vi "CAN通信实验.vi"() -> ()   [LabVIEW 2011]
uses:
  <vilib>/STM32_DriverVI_Interface_F4/CAN/Frame Stand_Extend_F4.ctl
  <vilib>/STM32_DriverVI_Interface_F4/CAN/Frame Data_Remote_F4.ctl
  <vilib>/STM32_DriverVI_Interface_F4/CAN/CAN Mode Set_F4.ctl
  <vilib>/STM32_DriverVI_Interface_F4/CAN/CAN Baud Rate_F4.ctl
  <vilib>/STM32_DriverVI_Interface_F4/CAN/CAN1_TX Pin Map_F4.ctl
  <vilib>/STM32_DriverVI_Interface_F4/CAN/CAN1_RX Pin Map_F4.ctl
  <vilib>/STM32_DriverVI_Interface_F4/CAN/CAN Filter_X Set_F4.ctl
  <vilib>/STM32_DriverVI_Interface_F4/CAN/Filter Enable_F4.ctl
  <vilib>/STM32_DriverVI_Interface_F4/CAN/CAN1 Init_F4.vi
  <vilib>/STM32_DriverVI_Interface_F4/CAN/CAN1 Filter Set_F4.vi
  <vilib>/STM32_DriverVI_Interface_F4/CAN/CAN1 Send Frame_F4.vi
  <vilib>/STM32_DriverVI_Interface_F4/CAN/CAN1 Frame Count_F4.vi
  <vilib>/STM32_DriverVI_Interface_F4/CAN/CAN1 Read Frame_F4.vi
panel:
  out "Send Success？":u16
  out "Init Success？":bool
  out "Frame Counts":u16
  out "Frame_Data":u8[][](array[numeric])
  in  "是否读取":bool
  in  "Frame Data or Remote":T1
  in  "Frame Stand or Extend":T2
  in  "Frame_ID":u32
  in  "数组长度":i32
  in  "点击发送":bool
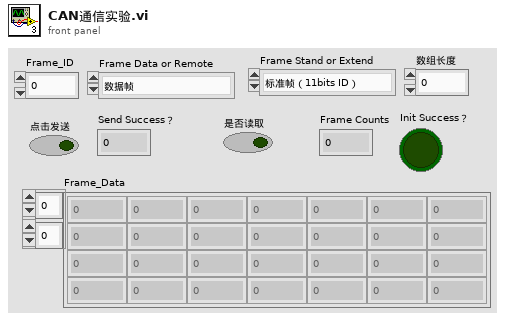
[diagram p1: front panel]
types:
  T1 = typedef "Frame Data_Remote_F4.ctl" = enum8{"数据帧", "远程帧"}
  T2 = typedef "Frame Stand_Extend_F4.ctl" = enum8{"标准帧（11bits ID）", "扩展帧（29bits ID）"}
  T3 = typedef "CAN Filter_X Set_F4.ctl" = enum8{"Filter_0", "Filter_1", "Filter_2", "Filter_3", "Filter_4", "Filter_5", "Filter_6", "Filter_7", "Filter_8", "Filter_9", "Filter_10", "Filter_11", "Filter_12", "Filter_13", "Filter_14", "Filter_15", "Filter_16", "Filter_17", "Filter_18", "Filter_19", "Filter_20", "Filter_21", "Filter_22", "Filter_23", "Filter_24", "Filter_25", "Filter_26", "Filter_27"}
  T4 = typedef "Filter Enable_F4.ctl" = enum8{"Disable", "Enable"}
  T5 = typedef "CAN1_RX Pin Map_F4.ctl" = u8
  T6 = typedef "CAN1_TX Pin Map_F4.ctl" = u8
  T7 = typedef "CAN Baud Rate_F4.ctl" = u16
  T8 = typedef "CAN Mode Set_F4.ctl" = enum8{"正常发送", "环回模式"}
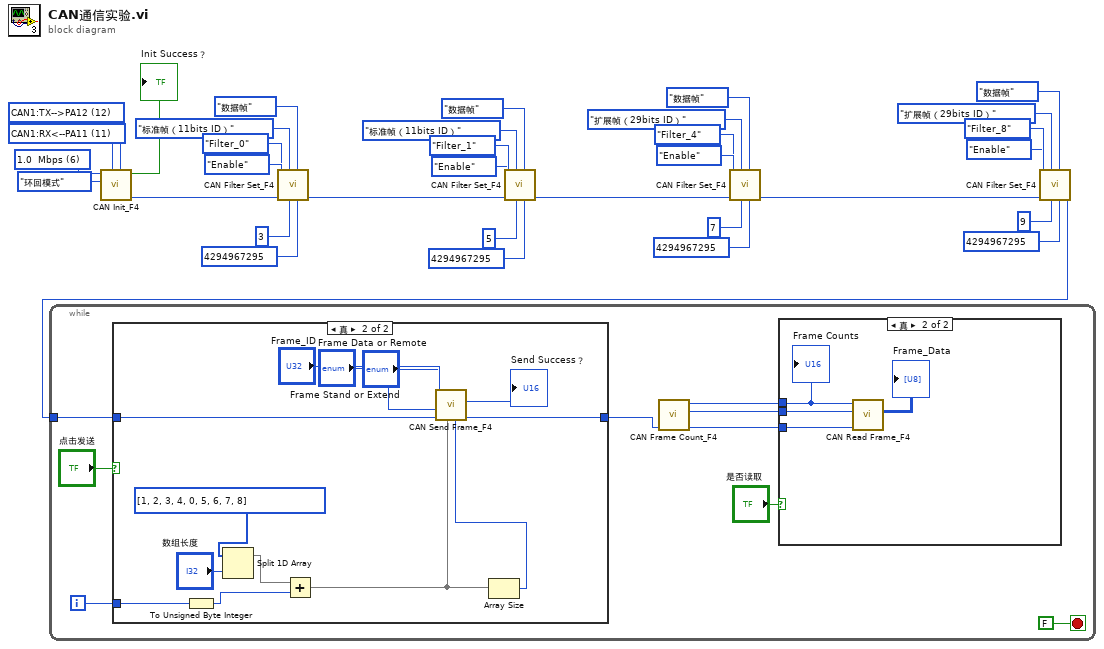
[diagram p0: block diagram]
diagram:
  w31 = T5 11 items=["CAN1:RX<--PA11"=11, "CAN1:RX<--PB8"=24, "CAN1:RX<--PD0"=48, "CAN1:RX<--PI9"=137] ("CAN1_RX Pin Map")
  w32 = T6 12 items=["CAN1:TX-->PA12"=12, "CAN1:TX-->PB9"=25, "CAN1:TX-->PD1"=49, "CAN1:TX-->PH13"=125] ("CAN1_TX Pin Map")
  w33 = T7 6 items=["1.0  Mbps"=6, "750 Kbps"=8, "600  Kbps"=10, "500  Kbps"=12, "400  Kbps"=15, "375  Kbps"=16, "300  Kbps"=20, "250  Kbps"=24, "200  Kbps"=30, "187.5Kbps"=32, "150   Kbps"=40, "125   Kbps"=48, "120   Kbps"=50, "100   Kbps"=60, "75     Kbps"=80, "60    Kbps"=100, "50    Kbps"=120, "40    Kbps"=150, "37.5  Kbps"=160, "30    Kbps"=200, "25    Kbps"=240, "20    Kbps"=300, "10    Kbps"=600, "5      Kbps"=1200] ("CAN Baud Rate")
  n1 = call-poly <vilib>:"CAN Init_F4.vi"("CAN1_RX Pin Map"=w31, "CAN1_TX Pin Map"=w32, "CAN Mode Setting"=CAN_Mode_Set_F4."环回模式", "CAN Baud Rate"=w33) -> ("err_out"=w30:u8, "Init Success？"=→"Init Success？":bool)  [unwired: 6 in]
  n2 = call-poly <vilib>:"CAN Filter Set_F4.vi"("ID_Mask"=u32 4294967295, "Frame Data or Remote"=Frame_Data_Remote_F4."数据帧", "Filter_ID"=u32 3, "Frame Stand or Extend"=Frame_Stand_Extend_F4."标准帧（11bits ID）", "err_in"=w30, "Filter Enable/Disable"=Filter_Enable_F4."Enable", "CAN Filter_X Setting"=CAN_Filter_X_Set_F4."Filter_0") -> ("err_out"=w5:u8)  [unwired: 4 in]
  n3 = call-poly <vilib>:"CAN Filter Set_F4.vi"("ID_Mask"=u32 4294967295, "Frame Data or Remote"=Frame_Data_Remote_F4."数据帧", "Filter_ID"=u32 5, "Frame Stand or Extend"=Frame_Stand_Extend_F4."标准帧（11bits ID）", "err_in"=w5, "Filter Enable/Disable"=Filter_Enable_F4."Enable", "CAN Filter_X Setting"=CAN_Filter_X_Set_F4."Filter_1") -> ("err_out"=w4:u8)  [unwired: 4 in]
  n4 = call-poly <vilib>:"CAN Filter Set_F4.vi"("ID_Mask"=u32 4294967295, "Frame Data or Remote"=Frame_Data_Remote_F4."数据帧", "Filter_ID"=u32 7, "Frame Stand or Extend"=Frame_Stand_Extend_F4."扩展帧（29bits ID）", "err_in"=w4, "Filter Enable/Disable"=Filter_Enable_F4."Enable", "CAN Filter_X Setting"=CAN_Filter_X_Set_F4."Filter_4") -> ("err_out"=w3:u8)  [unwired: 4 in]
  n5 = call-poly <vilib>:"CAN Filter Set_F4.vi"("ID_Mask"=u32 4294967295, "Frame Data or Remote"=Frame_Data_Remote_F4."数据帧", "Filter_ID"=u32 9, "Frame Stand or Extend"=Frame_Stand_Extend_F4."扩展帧（29bits ID）", "err_in"=w3, "Filter Enable/Disable"=Filter_Enable_F4."Enable", "CAN Filter_X Setting"=CAN_Filter_X_Set_F4."Filter_8") -> ("err_out"=w2:u8)  [unwired: 4 in]
  n6 = while {
    tunnel: w2 -> [w42]
    i -> [w41]
    stop <- FALSE stop-if-true
    n7 = case shown="真" "点击发送" {
      tunnel: w42 -> [_ w49]
      tunnel: w41 -> [_ w60]
      tunnel: [_ w52] -> w40
      frame False {
      }
      frame True {
        n8 = To Unsigned Byte Integer(number=w60) -> (unsigned 8bit integer=w59:u8)
        n9 = Split 1D Array(array=i32[] [1, 2, 3, 4, 0, 5, 6, 7, 8], index="数组长度") -> (first subarray=w57:i32[])  [unwired: 1 out]
        n10 = Add(x=w57, y=w59) -> (x+y=w50:i32[])
        n11 = Array Size(array=w50) -> (size(s)=w51:i32)
        n12 = call-poly <vilib>:"CAN Send Frame_F4.vi"("Data_Length"=w51, "Data[U8]"=w50, "err_in"=w49, "Frame Data or Remote"="Frame Data or Remote", "Frame Stand or Extend"="Frame Stand or Extend", "Frame_ID"="Frame_ID") -> ("err_out"=w52:u8, "Send Success？"=→"Send Success？":u16)  [unwired: 3 in, 1 out]
      }
    }
    n13 = call-poly <vilib>:"CAN Frame Count_F4.vi"("err_in"=w40) -> ("err_out"=w37:u8, "Buffer Counts"=w36:u16, "Frame Counts"=w35:u16)  [unwired: 8 in]
    n14 = case shown="真" "是否读取" {
      tunnel: w37 -> [_ w47]
      tunnel: w36 -> [_ w46]
      tunnel: w35 -> [_ w45]
      frame False {
      }
      frame True {
        n15 = call-poly <vilib>:"CAN Read Frame_F4.vi"("err_in"=w47, "CAN Buffer Size"=w46, "CAN Frame Counts"=w45) -> ("Frame_Data"=→"Frame_Data":u8[][])  [unwired: 6 in, 2 out]
        "Frame Counts" <- w45
      }
    }
  }
